vi "Ridders Zero Inner Part.vi"(0 "start/end/f(x)":T1 {"end" format="%.2f"; "start" format="%.2f"; "y value copy" format="%.2f"; "y value" format="%.2f"}, 1 "list of variables":i32[](array[numeric]), 2 "table":i32[][](array[numeric]), 3 "result":dbl[](array[numeric]) format="%.2f", 4 "accuracy":dbl format="%.2f", 5 "case":bool) -> (6 "y value":dbl format="%.2f", 7 "end":dbl format="%.2f", 8 "error":i32)   [LabVIEW 2020, in "NI_Gmath.lvlib"]
uses:
  <vilib>/gmath/NI_Gmath.lvlib
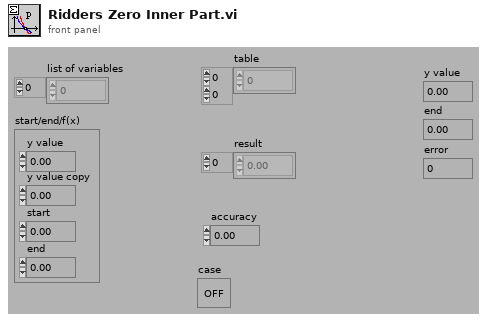
[diagram p1: front panel]
types:
  T1 = cluster{"y value":dbl, "y value copy":dbl, "start":dbl, "end":dbl}
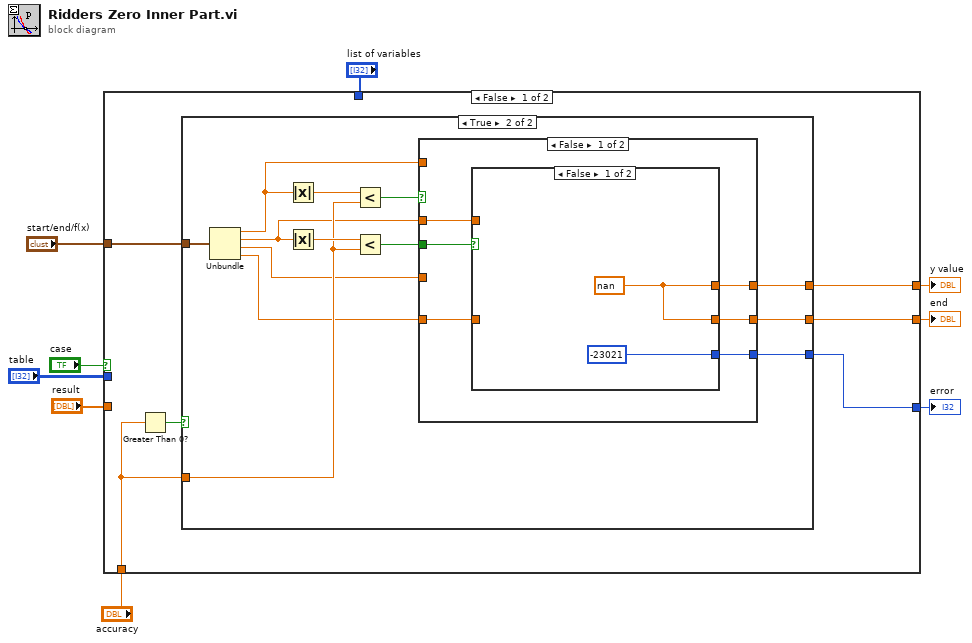
[diagram p0: block diagram]
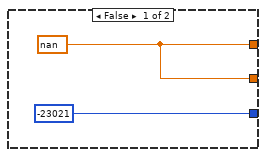
[diagram p2: hidden frame]
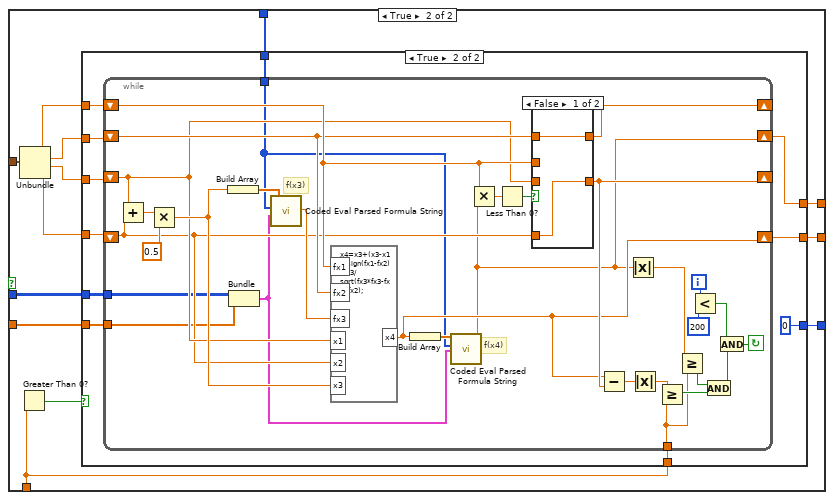
[diagram p5: hidden frame]
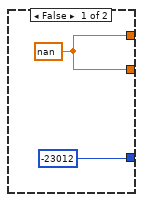
[diagram p6: hidden frame]
diagram:
  n1 = case shown="False" "case" {
    tunnel: [w12 w54] -> w2
    tunnel: "accuracy" -> [w10 w48]
    tunnel: [w13 w53] -> w4
    tunnel: [w14 w52] -> w5
    tunnel: "list of variables" -> [_ w51]
    tunnel: "table" -> [_ w50]
    tunnel: "result" -> [_ w49]
    tunnel: "start/end/f(x)" -> [w15 w47]
    frame False {
      n2 = Greater Than 0?(x=w10) -> (x > 0?=w11:bool)
      n3 = case shown="True" w11 {
        tunnel: w15 -> [_ w30]
        tunnel: w10 -> [_ w27]
        tunnel: [w16 w21] -> w14
        tunnel: [w16 w20] -> w13
        tunnel: [-23021 w18] -> w12
        frame False {
          w16 = nan ("y value copy")
        }
        frame True {
          n4 = Unbundle(w30) -> ("y value"=w25:dbl, "y value copy"=w22:dbl, "start"=w24:dbl, "end"=w23:dbl)
          n5 = Absolute Value(x=w25) -> (abs(x)=w29:dbl)
          n6 = Absolute Value(x=w22) -> (abs(x)=w28:dbl)
          n7 = Less?(x=w29, y=w27) -> (x < y?=w26:bool)
          n8 = Less?(x=w28, y=w27) -> (x < y?=w19:bool)
          n9 = case shown="False" w26 {
            tunnel: w25 -> [_ w42]
            tunnel: w24 -> [_ w41]
            tunnel: w23 -> [w32 _]
            tunnel: w22 -> [w34 _]
            tunnel: [w35 w42] -> w21
            tunnel: [w33 w41] -> w20
            tunnel: w19 -> [w36 _]
            tunnel: [w31 _] -> w18
            frame False {
              n10 = case shown="False" w36 {
                tunnel: [w38 w40] -> w35
                tunnel: w34 -> [_ w40]
                tunnel: [w38 w39] -> w33
                tunnel: w32 -> [_ w39]
                tunnel: [-23021 _] -> w31
                frame False {
                  w38 = nan ("y value copy")
                }
                frame True {
                }
              }
            }
            frame True {
            }
          }
        }
      }
    }
    frame True {
      n11 = Greater Than 0?(x=w48) -> (x > 0?=w55:bool)
      n12 = Unbundle(w47) -> ("y value"=w43:dbl, "y value copy"=w44:dbl, "start"=w45:dbl, "end"=w46:dbl)
      n13 = case shown="True" w55 {
        tunnel: w48 -> [_ w68]
        tunnel: w43 -> [_ w67]
        tunnel: w44 -> [_ w66]
        tunnel: w45 -> [_ w65]
        tunnel: w46 -> [_ w64]
        tunnel: [-23012 0] -> w54
        tunnel: [w56 w62] -> w53
        tunnel: [w56 w61] -> w52
        tunnel: w51 -> [_ w60]
        tunnel: w50 -> [_ w59]
        tunnel: w49 -> [_ w58]
        frame False {
          w56 = nan
        }
        frame True {
          n14 = while {
            tunnel: w58 -> [w70]
            tunnel: w59 -> [w72]
            tunnel: w60 -> [w71]
            tunnel: w68 -> [w82]
            shift-left: w66 -> [w93]
            shift-right: [w69] -> w61
            shift-left: w67 -> [w95]
            shift-right: [w94] -> _
            shift-left: w64 -> [w83]
            shift-right: [w81] -> w62
            shift-left: w65 -> [w84]
            shift-right: [w92] -> _
            i -> [w80]
            stop <- w77 continue-if-true
            # "f(x4)"
            # "f(x3)"
            n15 = Add(x=w84, y=w83) -> (x+y=w98:dbl)
            n16 = Multiply(x=w98, y=0.5) -> (x*y=w85:dbl)
            n17 = Build Array(w85) -> (w75:dbl[])
            n18 = Bundle("table"=w72, "result"=w70) -> (w74:cluster{"table":i32[][], "result":dbl[]})  [unwired: 1 in]
            n19 = call <vilib>:"Coded Eval Parsed Formula String.vi"("Parsed Formula"=w74, "Variables"=w71, "X Values"=w75) -> ("y value"=w86:dbl)  [unwired: 1 in, 1 out]
            n20 = formula code="x4=x3+(x3-x1)*sign(fx1-fx2)*fx3/sqrt(fx3*fx3-fx1*fx2);"("fx1"=w95, "fx2"=w93, "fx3"=w86, "x1"=w84, "x2"=w83, "x3"=w85) -> ("x4"=w81:dbl)
            n21 = Build Array(w81) -> (w73:dbl[])
            n22 = call <vilib>:"Coded Eval Parsed Formula String.vi"("Parsed Formula"=w74, "Variables"=w71, "X Values"=w73) -> ("y value"=w69:dbl)  [unwired: 1 in, 1 out]
            n23 = Multiply(x=w95, y=w69) -> (x*y=w97:dbl)
            n24 = Less Than 0?(x=w97) -> (x < 0?=w96:bool)
            n25 = case shown="False" w96 {
              tunnel: w84 -> [_ w103]
              tunnel: [w101 w103] -> w92
              tunnel: w83 -> [w101 _]
              tunnel: w95 -> [_ w102]
              tunnel: [w100 w102] -> w94
              tunnel: w93 -> [w100 _]
              frame False {
              }
              frame True {
              }
            }
            n26 = Subtract(x=w81, y=w92) -> (x-y=w90:dbl)
            n27 = Absolute Value(x=w69) -> (abs(x)=w89:dbl)
            n28 = Absolute Value(x=w90) -> (abs(x)=w91:dbl)
            n29 = Greater Or Equal?(x=w91, y=w82) -> (x >= y?=w87:bool)
            n30 = Greater Or Equal?(x=w89, y=w82) -> (x >= y?=w88:bool)
            n31 = Less?(x=w80, y=200) -> (x < y?=w78:bool)
            n32 = And(x=w88, y=w87) -> (x .and. y?=w76:bool)
            n33 = And(x=w78, y=w76) -> (x .and. y?=w77:bool)
          }
        }
      }
    }
  }
  "y value" <- w5
  "end" <- w4
  "error" <- w2
